vi "Zoom.vi"(11 "IntGraph Refnum":refnum<vi>) -> ()   [LabVIEW 2014]
panel:
  out "Focal Spot":dbl[][](graph)
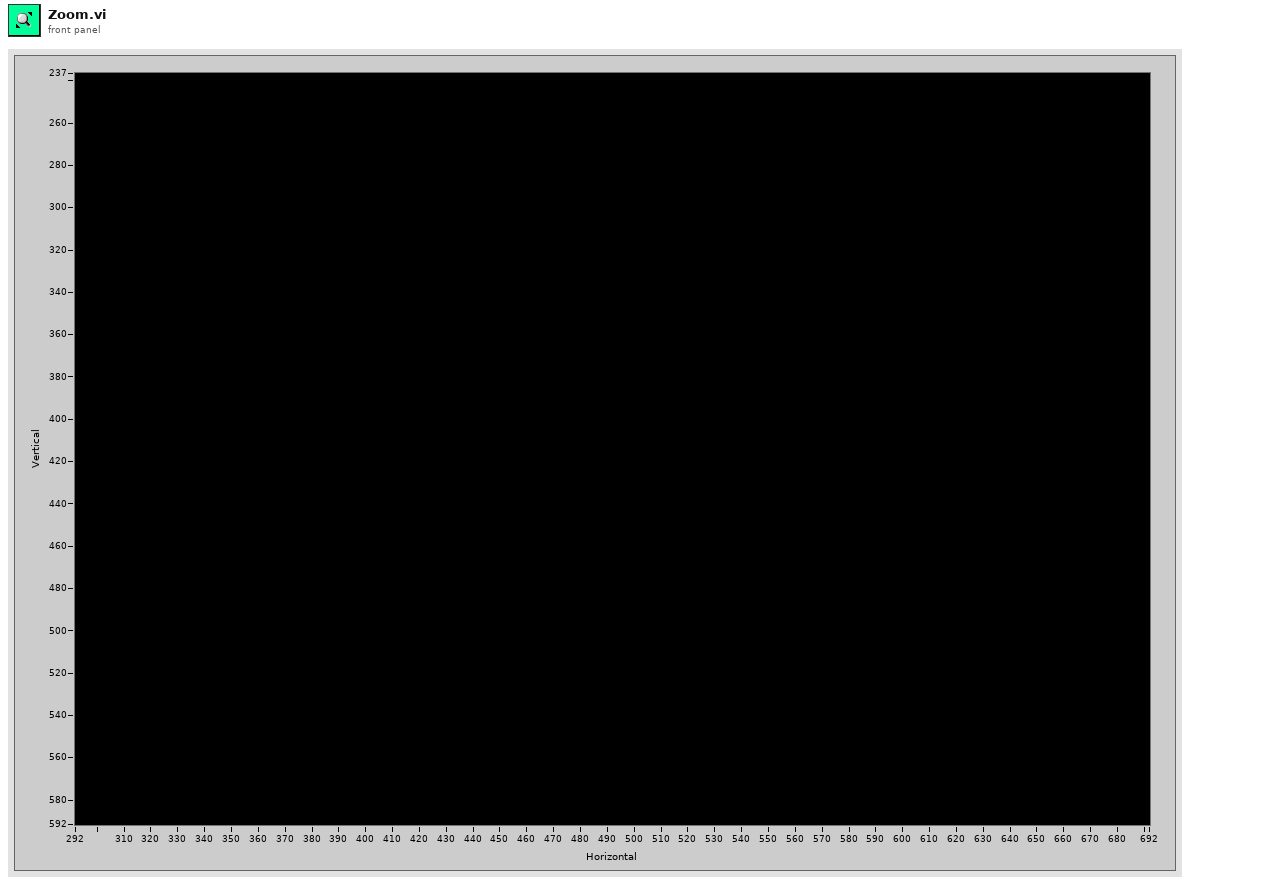
[diagram p1: front panel]
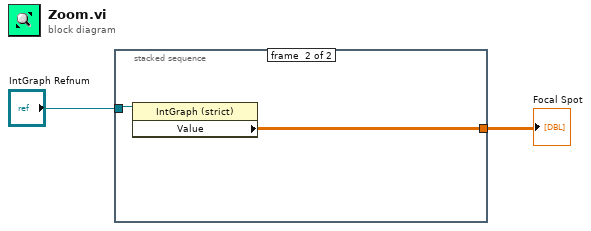
[diagram p0: block diagram]
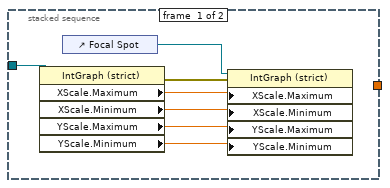
[diagram p2: hidden frame]
diagram:
  n1 = stacked-sequence {
    tunnel: [_ w11] -> w2
    tunnel: "IntGraph Refnum" -> [w9 w10]
    frame #0 {
      n2 = property class="IntGraph (strict)"(reference=w9) -> (error out=w7:errorcluster, "XScale.Maximum"=w6:dbl, "XScale.Minimum"=w5:dbl, "YScale.Maximum"=w4:dbl, "YScale.Minimum"=w3:dbl)  [unwired: 1 in, 1 out]
      n3 = control-ref of="Focal Spot"() -> (w8:refnum<vi>)
      n4 = property class="IntGraph (strict)"(reference=w8, error in=w7, "XScale.Maximum"=w6, "XScale.Minimum"=w5, "YScale.Maximum"=w4, "YScale.Minimum"=w3) -> ()  [unwired: 2 out]
    }
    frame #1 {
      n5 = property class="IntGraph (strict)"(reference=w10) -> ("Value"=w11:dbl[][])  [unwired: 1 in, 2 out]
    }
  }
  "Focal Spot" <- w2
